vi "GoToTest.vi"(8 "command\nenum":T1, 9 "Robot In":T2, 11 "GoTo point":dbl[](array[numeric])=[0.0, 0.0, 0.0]) -> (1 "Robot Out":T2)   [LabVIEW 2016]
uses:
  Core/AI Robot.ctl
  Intel/Functions Enum.ctl
  Intel/Command Enum.ctl
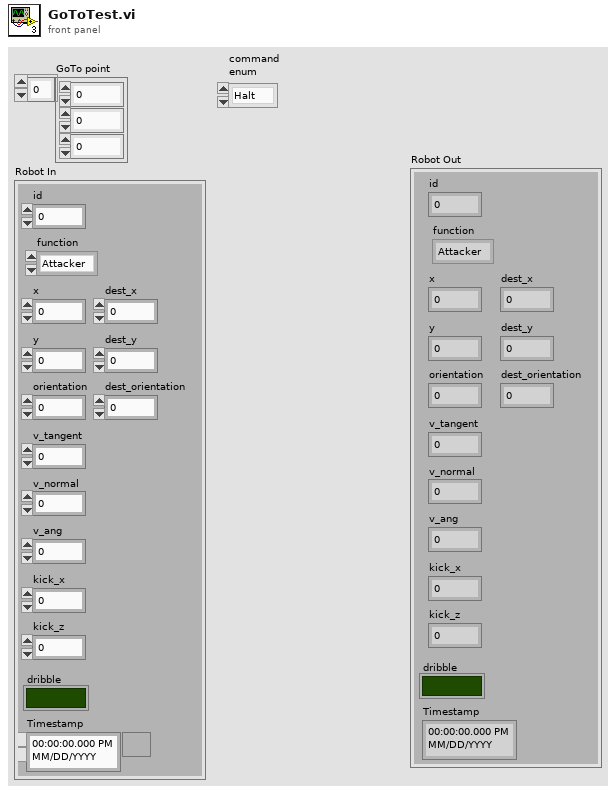
[diagram p1: front panel]
types:
  T1 = typedef "Command Enum.ctl" = enum16{"Halt", "Stop", "Force Start", "PKA Normal Start", "Prepare Kickoff Ally", "PKE Normal Start", "Prepare Kickoff Enemy", "Prepare Penalty Ally", "PPA Normal Start", "Prepare Penalty Enemy", "PPE Normal Start", "Direct Free Enemy", "Direct Free Ally", "Indirect Free Enemy", "Indirect Free Ally", "Timeout Enemy", "Timeout Ally", "Goal Enemy", "Goal Ally", "Ball Placement Enemy", "Ball Placement Ally", "None"}
  T2 = typedef "AI Robot.ctl" = cluster{"id":u32, "function":T3, "x":dbl, "y":dbl, "orientation":dbl, "v_tangent":dbl, "v_normal":dbl, "v_ang":dbl, "kick_x":dbl, "kick_z":dbl, "dribble":bool, "Timestamp":timestamp, "dest_x":dbl, "dest_y":dbl, "dest_orientation":dbl}
  T3 = typedef "Functions Enum.ctl" = enum16{"Attacker", "Goalie", "Defender", "Striker", "Goto 0", "Dummy", "ZigZag"}
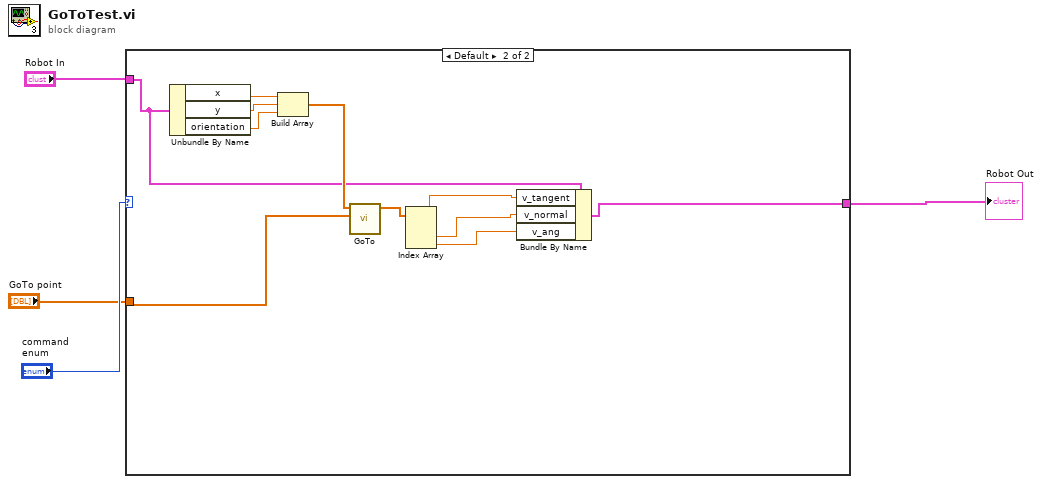
[diagram p0: block diagram]
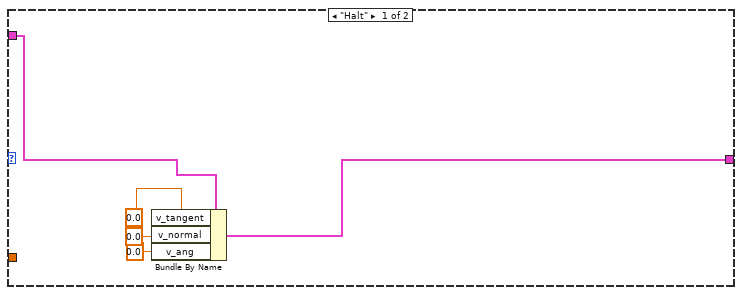
[diagram p2: hidden frame]
diagram:
  n1 = case shown="Default" "command\nenum" {
    tunnel: [w5 w10] -> w3
    tunnel: "Robot In" -> [w9 w15]
    tunnel: "GoTo point" -> [_ w20]
    frame "Halt" {
      n2 = Bundle By Name(cluster=w9, "v_tangent"=0.0, "v_normal"=0.0, "v_ang"=0.0) -> (w5:T2)
    }
    frame Default {
      n3 = Unbundle By Name(w15) -> ("x"=w19:dbl, "y"=w18:dbl, "orientation"=w17:dbl)
      n4 = Build Array(w19, w18, w17) -> (w16:dbl[])
      n5 = call "GoTo.vi"("Target"=w20, "Position"=w16) -> ("Output\nVelocity"=w14:dbl[])  [unwired: 8 in, 1 out]
      n6 = Index Array(array=w14) -> (element #1=w13:dbl, element #2=w12:dbl, element #3=w11:dbl)  [unwired: 3 in]
      n7 = Bundle By Name(cluster=w15, "v_tangent"=w13, "v_normal"=w12, "v_ang"=w11) -> (w10:T2)
    }
  }
  "Robot Out" <- w3
